vi "Power Off.vi"(8 "error in (no error)":errorcluster, 11 "Dual Fan in":refnum<class "Dual Fan.lvclass">) -> (0 "error out":errorcluster, 3 "Dual Fan out":refnum<class "Dual Fan.lvclass">)   [LabVIEW 2012, in "Dual Fan.lvlib" / "Dual Fan.lvclass"]
uses:
  Dual Fan.lvclass
  Dual Fan.lvclass/Dual Fan.ctl
  Simulation/Simulation Data_Global.vi
  Simulation/Simulation.lvlib
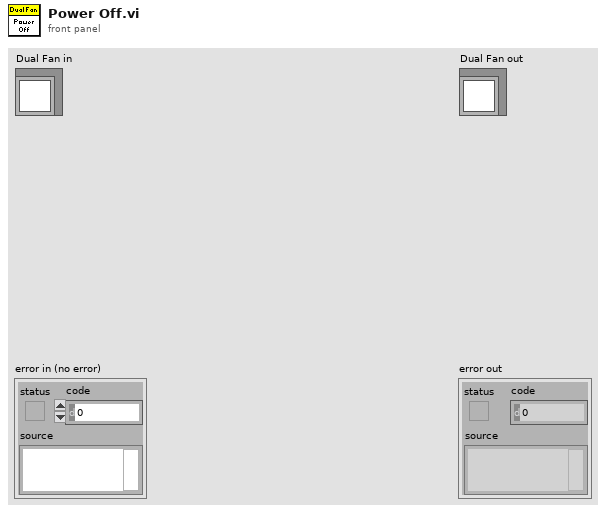
[diagram p1: front panel]
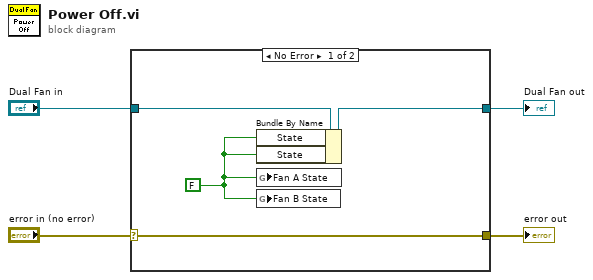
[diagram p0: block diagram]
diagram:
  n1 = case shown="No Error" "error in (no error)" {
    selector: "error in (no error)" -> [w8 w10]
    tunnel: [w8 w10] -> w3
    tunnel: [w6 w9] -> w1
    tunnel: "Dual Fan in" -> [w7 w9]
    frame No Error {
      w5 = FALSE ("Fan A State")
      n2 = Bundle By Name(cluster=w7, "State"=w5, "State"=w5) -> (w6:refnum<class "Dual Fan.lvclass">)
      n3 = global write "Simulation Data_Global.vi" "Fan A State"(w5) -> ()
      n4 = global write "Simulation Data_Global.vi" "Fan B State"(w5) -> ()
    }
    frame Error {
    }
  }
  "error out" <- w3
  "Dual Fan out" <- w1
